vi "Find Commands.vi"(11 "TargetItem in":refnum<vi>) -> ()   [LabVIEW 2020]
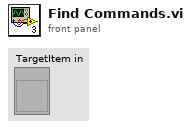
[diagram p1: front panel]
types:
  T1 = typedef "imagedata.ctl" = cluster{"image type":i32, "image depth":i32, "image":u8[], "mask":u8[], "colors":u32[], "Rectangle":cluster{"left":i16, "top":i16, "right":i16, "bottom":i16}}
  T2 = cluster{"Name":string, "CPTM.DataType":variant, "Get All Control Values Variant":cluster{"Name":string, "Variant Data":variant}[], "Color 256":T1, "Subsystem Color":u32}[]
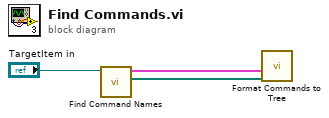
[diagram p0: block diagram]
diagram:
  n1 = call "Find Command Names.vi"("TargetItem in"="TargetItem in") -> ("Paths"=w1:path[], "Command Info"=w2:T2)  [unwired: 9 in]
  n2 = call "Format Commands to Tree.vi"("Paths"=w1, "Command Info"=w2) -> ()  [unwired: 8 in, 2 out]
